vi "Run.vi"(8 "Error In":errorcluster, 10 "Frame Count":u64, 11 "Animation In":refnum<class "Animation.lvclass">) -> (0 "Error Out":errorcluster, 2 "Display Elements":refnum<class "Display Element.lvclass">[](array[class]), 3 "Animation Out":refnum<class "Animation.lvclass">)   [LabVIEW 2021, in "Animation.lvclass"]
uses:
  Animation.lvclass
  Display Element/Display Element.lvclass
  Animation.lvclass/Animation.ctl
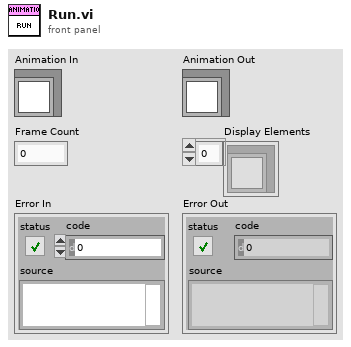
[diagram p1: front panel]
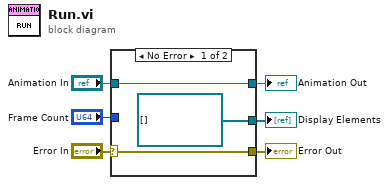
[diagram p0: block diagram]
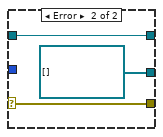
[diagram p2: hidden frame]
diagram:
  n1 = case shown="No Error" "Error In" {
    selector: "Error In" -> [w9 w11]
    tunnel: "Animation In" -> [w8 w12]
    tunnel: [w9 w11] -> w4
    tunnel: [w8 w12] -> w3
    tunnel: [refnum<class "Display Element.lvclass">[] [] ("Display Elements") refnum<class "Display Element.lvclass">[] [] ("Display Elements")] -> w2
    tunnel: "Frame Count" -> [_ _]
    frame No Error {
    }
    frame Error {
    }
  }
  "Animation Out" <- w3
  "Error Out" <- w4
  "Display Elements" <- w2
